vi "CloseFile.vi"(8 "error in (no error)":errorcluster, 11 "ReadOnly in":refnum<class "ReadOnly.lvclass">) -> (0 "error out":errorcluster)   [LabVIEW 2021, in "ReadOnly.lvclass"]
uses:
  ReadOnly.lvclass
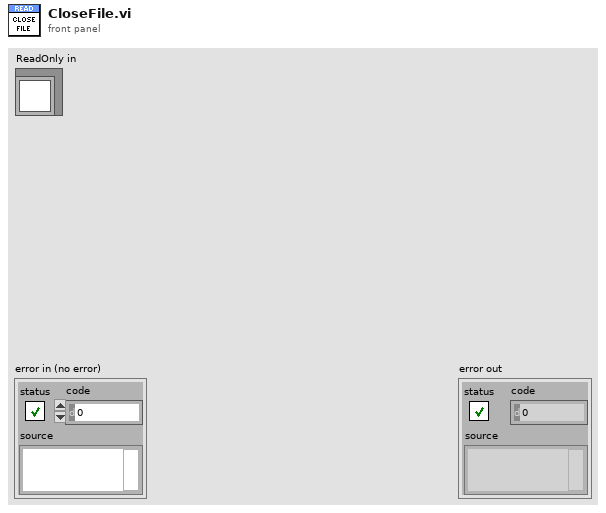
[diagram p1: front panel]
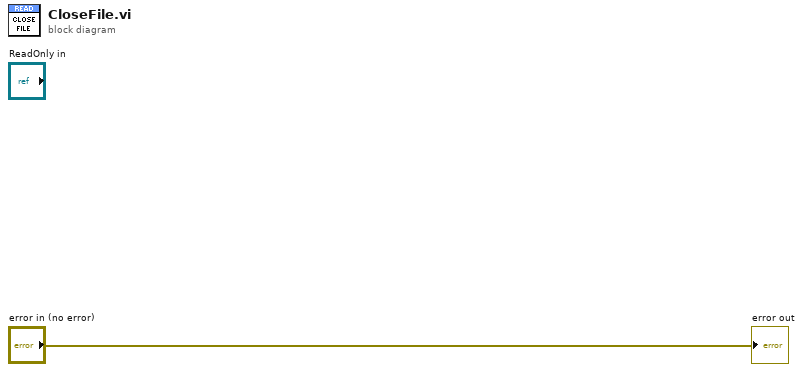
[diagram p0: block diagram]
diagram:
  "error out" <- "error in (no error)"
